vi "UpdateTargetDistances.vi"   [LabVIEW 2011]
uses:
  Robot Global Data.vi
types:
  T1 = cluster{"Position":cluster{"X":dbl, "Y":dbl}, "Distance (ft)":dbl}[]
  T2 = cluster{"Position":cluster{"X":dbl, "Y":dbl}, "Distance (ft)":dbl}
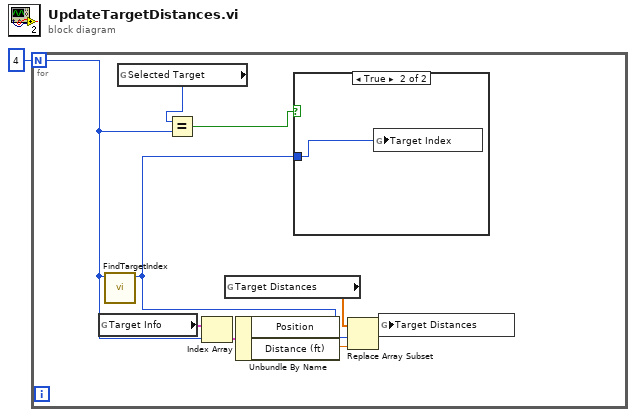
[diagram p0: block diagram]
diagram:
  n1 = for {
    N: 4 -> [w4]
    n2 = global read "Robot Global Data.vi" "Target Info"() -> (w8:T1)
    n3 = call "FindTargetIndex.vi"("Selected Target"=w4) -> ("Target Index"=w2:i32)  [unwired: 10 in]
    n4 = global read "Robot Global Data.vi" "Selected Target"() -> (w5:i32)
    n5 = Equal?(x=w5, y=w4) -> (x = y?=w3:bool)
    n6 = Index Array(array=w8, index=w4) -> (element=w7:T2)
    n7 = global read "Robot Global Data.vi" "Target Distances"() -> (w10:dbl[])
    n8 = Unbundle By Name(w7) -> ("Distance (ft)"=w6:dbl)  [unwired: 1 out]
    n9 = case shown="True" w3 {
      tunnel: w2 -> [_ w11]
      frame False {
      }
      frame True {
        n10 = global write "Robot Global Data.vi" "Target Index"(w11) -> ()
      }
    }
    n11 = Replace Array Subset(array=w10, new element=w6, index=w2) -> (w9:dbl[])
    n12 = global write "Robot Global Data.vi" "Target Distances"(w9) -> ()
  }
